vi "wsi1.vi"() -> ()   [LabVIEW 2018]
uses:
  <vilib>/addons/Modulation/Analog/support/mod_Set Error Source.vi
  <vilib>/addons/Modulation/Digital/Support/Common/Validators/mod_AWGN Validate.vi
  <vilib>/addons/Modulation/Digital/Impairments/subVIs/mod_createSeeds.vi
  <vilib>/addons/Modulation/Digital/Support/Common/Validators/mod_Validate Samples Per Symbol.vi
  <vilib>/addons/Modulation/Analog/support/Validators/mod_Validate Complex Waveform.vi
  <vilib>/addons/Modulation/Analog/support/Validators/mod_WFErrorHandler.vi
  <vilib>/addons/Modulation/Digital/General/MT Generate PSK System Parameters(M).vi
  <vilib>/addons/Modulation/Digital/Support/Common/Validators/mod_Generate Filter Coefficients Validate.vi
  <vilib>/addons/Modulation/Digital/General/subVIs/mod_Generate Filter Coefficients.vi
  <vilib>/addons/Modulation/Digital/General/subVIs/mod_Generate Bits PN Sequence.vi
  <vilib>/Analysis/1siggen.llb/Gaussian White Noise (obs 90).vi
  <vilib>/addons/Modulation/niDMT.lvlib
panel:
  in  "autoscale":bool
  in  "stop":bool
  in  "pulse shaping filter":T1(ring)=enum."Root Raised Cos"
  in  "Noise Impairments":dbl(slide)=30.0 scale=0.0..100.0
  in  "M-PSK":i32(ring)=8 items=["4"=4, "8"=8, "16"=16, "32"=32]
  out "Constellation Plot":T2(graph)=[{"constellation"=[-0.39322774166480234, 0.9183146787671056, -0.40832338248208166, -0.38582449870261126, 0.3883539290960832, 0.3795255778951412, 0.3391931892211584, -0.404166356503105, 0.8770645695214075, 0.908012528356732, -0.40350648917432347, -0.3900703444457665, 0.3982891183517766, 0.4078034366046158, 0.9553544838279117, -0.3755905725981982, 0.8777236495651515, 0.9432196522594848, 0.3780170589478005, -0.8897154453948038, 0.38960218431345633, -0.9660260927981917, 0.9180192288796393, 0.38626663120651866, 0.9356807404587103, -0.43062910837213464, 0.9336768818408142, -0.36939057337864706, 0.9500976391200191, -0.9344273698827297, 0.9287782284181648, -0.3838044438259214, 0.9097324398288045, 0.40096098663389784, -0.9168611190862982, 0.8872499130805949, 0.39576755530907615, -0.39736171842545376, -0.3982036697877337, 0.9639467434400133, 0.928478338730628, -0.9784713409136321, -0.404209697626999, 0.9255365386679252, 0.3563945363973958, 0.9410821960139222, -0.39200275806886337, 0.37316817129413854, 0.3707703792663171, -0.9190126834545177, -0.8989722948561384, 0.37590466197124406, -0.9539018667097078, 0.38170683383925824, 0.9162485880176054, -0.4610820448809754, 0.400034964231639, 0.9353231133425658, 0.902843039076622, -0.9131259844266787, -0.8886588059925667, 0.9479089649017637, -0.9038240228366312, 0.9428600359514282, 0.37125517874574004, 0.3976034844476846, 0.9908858043950586, -0.3918288246994119, 0.3561171825179303, -0.37305696824280954, 0.3814388799800192, -0.9412695704675936, -0.9301299947614053, -0.9683088822641316, -0.41077384261534056, -0.91113940207828, 0.9157980695922476, -0.8985409896225468, 0.32520003642858564, 0.904677180302555, 0.4199800599119881, 0.42170094290625776, -0.9403650565488012, -0.3735576880363529, -0.9604640725126443, -0.38170072894831397, -0.3692427902129988, 0.9692957282923731, -0.9115231822240809, -0.37981008528810356, 0.893486263853844, 0.9183965084935307, -0.37317430329662604, -0.9477116518222086, 0.9363344844465349, -0.37568715480480186, 0.894481077128131, -0.33215856645075925, -0.370105437085946, 0.9106253170668458, -0.8940744549927242, -0.3730162083433324, 0.3648524069495202, -0.9370323640820335, 0.39057992510472733, 0.3846794209195827, -0.9206135190097646, 0.9027845575240497, 0.8964264373458389, 0.38355295871088024, -0.3923606769062117, 0.9119453534901103, -0.3606253498724758, 0.8951824410447927, -0.9137445050115693, -0.4221123010713116, -0.38148184935595386, -0.40135884258831317, 0.37081487521698364, -0.9056737486669103, -0.9171166903310819, 0.9188814190590084, -0.886122882584363, 0.9173035920647417, 0.890341274676089, 0.40042927886514185, 0.34624386655619144, -0.4005189587598808, -0.37369233726172096, -0.3944826203694957, -0.9047062734940368, 0.38519673798677856, -0.370956195985644, -0.9005378061394372, -0.9428927398845177, -0.3917275570901477, -0.9177752615984011, 0.3651979881683026, -0.3724090746812553, -0.9310012999774543, -0.4234652879832877, -0.33125515596470556, -0.37359785279607743, 0.3658517972217536, 0.38918357750250415, 0.9189027923835421, -0.9048124953315838, 0.942229338715018, 0.930093948596154, -0.3932104754075415, -0.9137631801841072, -0.3906800265160916, 0.8911993175456597, -0.36431889648293164, -0.9405996374242932, 0.4283265501762037, -0.9088485250892261, 0.3655560533408721, 0.38900082599021163, 0.3777238638853494], "oversampled data"=[0.9463096148397003, 0.33506866281920894, -0.9446033133340977, -0.9156199212317229, -0.8853463145803698, -0.9494424420181075, -0.9451139376818354, -0.9034596446685559, 0.3744111108058542, 0.3572404678439043, 0.9171206593064269, 0.9609091479875221, 0.937768343063285, -0.9422877481286908, -0.368600409468377, 0.9129237365738408, 0.31900696673194906, 0.42323694407222145, 0.9191482420186188, 0.3674481406094202, 0.9270845037922253, -0.41197434621206, -0.3844269297281987, 0.9219923803383505, -0.3996928183504703, 0.891949665165261, -0.41214943136295046, 0.9108939618295051, 0.3192019606883094, 0.3711053280053422, 0.3833664318720858, -0.906540726227132, 0.389060177928031, -0.9112937649466583, 0.3663420060225401, -0.38172194821683036, -0.9148305759918348, -0.9049425802203815, -0.9014520007052044, 0.38676659106578104, -0.3678657176882371, 0.39827741084625073, 0.9295090378831258, -0.3743315357204549, -0.8881003024856062, 0.40919730097603774, -0.9144230209512562, 0.9272112215032523, -0.9340593007543905, -0.4180073399318941, 0.3737628645677372, -0.9207654340258427, -0.35024575424408094, 0.9424214865929558, -0.3685222634786592, -0.9481547299664241, -0.9082207264478568, 0.35641522054932717, -0.33566823263279205, -0.38287466504945505, 0.36487924474235645, -0.4070999956325476, -0.37270707645349377, 0.40674715012166024, -0.922336060263489, -0.9014589201773306, -0.3444903803741438, -0.9623111690420606, 0.9285088915542266, -0.9422666928068593, 0.9268620371561562, 0.36191119218242385, -0.3837828811665712, -0.37270874268828824, 0.9184772521939574, -0.4004925359918762, 0.39596083370254376, 0.3770594251709337, -0.9046850565699176, 0.36596185169113377, 0.903342323213868, 0.9816028006559513, -0.3738144865554587, -0.9162121916394916, -0.41780464730481065, 0.9329802433071399, -0.9119254544133856, 0.3677436309457829, -0.37908204260355116, 0.9338883592942152, 0.38604359647323594, 0.4072846810170729, -0.9091657676345222, 0.3485041296986709, -0.361978137733223, -0.9267599286737814, 0.38903001551475913, -0.9025538983311643, 0.8999866217246261, -0.38171678403575093, -0.36819596197125143, -0.9357962610551767, -0.9322588086357637, 0.4147593852424159, -0.9296076176838902, -0.9316993844695177, -0.42883574011674225, 0.3896284958599367, -0.3535366162765058, -0.9117067894884218, 0.9554215703618354, 0.3874411783216424, 0.9212148734531419, 0.40291191098343526, -0.3805018304847159, -0.9087880814762439, -0.893681944453442, 0.972515898155951, -0.9143359583780245, -0.40532730056400507, -0.40870878544746264, -0.3806799251745927, -0.42052822773833665, -0.3837946859923954, -0.3519758533282975, -0.9194192968508207, 0.9396675771352186, -0.9374993763285927, 0.9172423798083785, 0.9175432355261142, -0.39890405383963423, -0.9158961357114441, 0.9209459512869621, 0.39577867677617407, 0.3618437914915072, 0.9462589734113327, 0.39955558499719684, -0.8991422352149865, 0.9474371495806615, -0.38497048804316303, 0.952071946877719, 0.9400061555632612, -0.9238791502699514, -0.9039914036164279, 0.9428084417673319, -0.4177928177003888, 0.40136932282294474, -0.4313109136414577, -0.37607058205614574, -0.9260285446809805, -0.3864404530502494, -0.9149193379336107, 0.38228607283424176, 0.9231694399506111, 0.36444985608249686, 0.8807909993150091, 0.4031790283255047, -0.9531656871658418, 0.9128903778214659, 0.9124141383796133]}, {"constellation"=array[2560 elements], "oversampled data"=array[2560 elements]}]
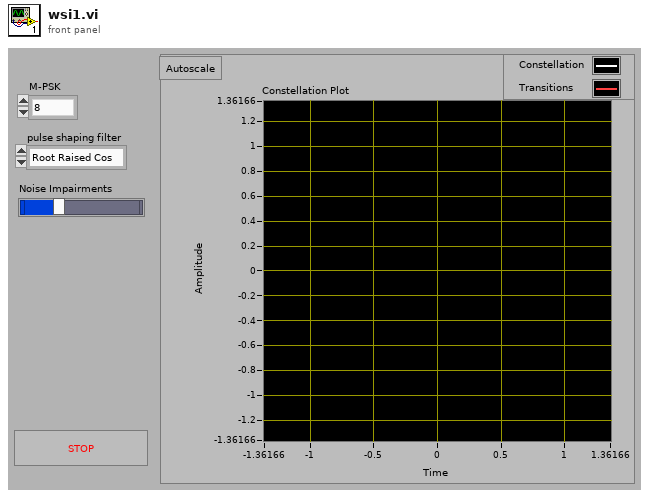
[diagram p1: front panel]
types:
  T1 = enum16{"none", "Raised Cosine", "Root Raised Cos"}
  T2 = cluster{"constellation":dbl[], "oversampled data":dbl[]}[]
  T3 = enum16{"FSK", "PSK", "QAM", "MSK", "PAM", "ASK", "CPM"}
  T4 = cluster{"samples per symbol (16)":i32, "symbol map":cdb[], "differential PSK":enum16{"disable", "enable"}, "PSK type":u16}
  T5 = typedef "niAMT.lvlib/Complex Data Waveform.ctl" = cluster{"t0":dbl, "dt":dbl, "Y":cdb[]}
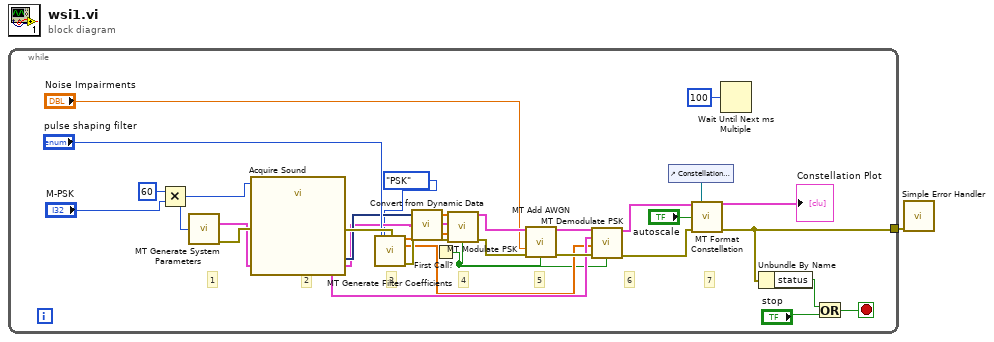
[diagram p0: block diagram]
diagram:
  n1 = while {
    tunnel: [w25] -> w1
    stop <- w26 stop-if-true
    # "7"
    # "6"
    # "5"
    # "4"
    # "3"
    # "2"
    # "1"
    n2 = Multiply(x=60, y="M-PSK") -> (x*y=w14:i32)
    n3 = call-poly <vilib>:"MT Generate System Parameters.vi"("differential PSK"=w14) -> ("PSK system parameters"=w7:T4, "error out"=w20:errorcluster)  [unwired: 12 in, 1 out]
    n4 = call "Acquire Sound"("Device"=w14, "error in (no error)"=w20) -> ("Data"=w16:dynamicdata, "error out"=w19:errorcluster)  [unwired: 16 in]
    n5 = call <vilib>:"MT Generate Filter Coefficients.vi"("modulation type"=T3."PSK", "pulse shaping samples per symbol (16)"="pulse shaping filter", "error in (no error)"=w19) -> ("pulse shaping filter coefficients"=w13:dbl[], "matched filter coefficients"=w6:dbl[], "error out"=w17:errorcluster)  [unwired: 10 in]
    n6 = call "Convert from Dynamic Data"("Dynamic Data Type"=w16) -> ("Array"=w15:dbl[])  [unwired: 3 in]
    n7 = First Call?() -> (First Call?: T/F=w5:bool)
    n8 = call <vilib>:"MT Modulate PSK.vi"("input bit stream"=w15, "PSK system parameters"=w7, "pulse shaping filter coefficients"=w13, "error in (no error)"=w17, "reset? (T)"=w5) -> ("output complex waveform"=w11:T5, "error out"=w12:errorcluster)  [unwired: 8 in, 1 out]
    n9 = call <vilib>:"MT Add AWGN.vi"("input complex waveform"=w11, "Eb/N0 (10 dB)"="Noise Impairments", "error in (no error)"=w12, "reset? (T)"=w5) -> ("output complex waveform"=w8:T5, "error out"=w9:errorcluster)  [unwired: 9 in, 1 out]
    n10 = call <vilib>:"MT Demodulate PSK.vi"("input complex waveform"=w8, "PSK system parameters"=w7, "matched filter coefficients"=w6, "error in (no error)"=w9, "reset? (T)"=w5) -> ("recovered complex waveform"=w3:T5, "error out"=w4:errorcluster)  [unwired: 6 in, 3 out]
    n11 = control-ref of="Constellation Plot"() -> (w29:refnum<vi>)
    n12 = call <vilib>:"MT Format Constellation.vi"("waveform"=w3, "constellation reference"=w29, "autoscale"="autoscale", "error in (no error)"=w4) -> ("constellation graph"=→"Constellation Plot":T2, "error out"=w25:errorcluster)  [unwired: 10 in]
    n13 = Wait Until Next ms Multiple(millisecond multiple=u32 100) -> ()  [unwired: 1 out]
    n14 = Unbundle By Name(w25) -> ("status"=w27:bool)
    n15 = Or(x=w27, y="stop") -> (x .or. y?=w26:bool)
  }
  n16 = call <vilib>:"Simple Error Handler.vi"("error in (no error)"=w1) -> ()  [unwired: 4 in, 5 out]
